vi "Handle timeline menu options.vi"(6 "Xinformation In":T2, 7 "Waveform Ref in":T1, 9 "ItemTag":string, 11 "Timeline Ref in":T4) -> (0 "error out":errorcluster, 3 "Timeline Ref out":T4, 4 "Xinformation Out":T2)   [LabVIEW 2020, in "XGrapher.xctl"]
uses:
  XGrapher.xctl
  Typedefs/Xctrl-Timeline graph ref.ctl
  Typedefs/Xinformation.ctl
  Typedefs/Xcrtl-Click Operation.ctl
  Typedefs/Xctrl-Waveform graph ref.ctl
  Typedefs/Registered event names enum.ctl
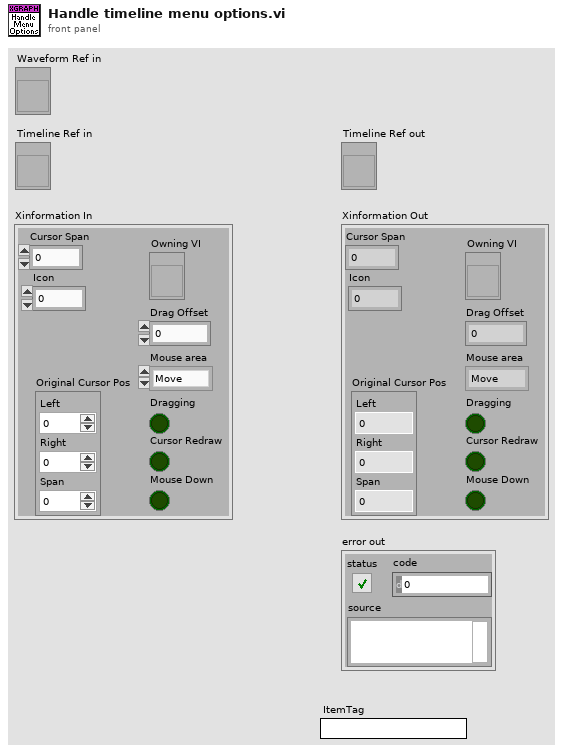
[diagram p1: front panel]
types:
  T1 = typedef "XGrapher.xctl/Xctrl-Waveform graph ref.ctl" = refnum<vi>
  T2 = typedef "XGrapher.xctl/Xinformation.ctl" = cluster{"Cursor Span":dbl, "Icon":u16, "Mouse Down":bool, "Owning VI":refnum<vi>, "Mouse area":T3, "Dragging":bool, "Drag Offset":dbl, "Original Cursor Pos":cluster{"Left":dbl, "Right":dbl, "Span":dbl}, "Cursor Redraw":bool}
  T3 = typedef "XGrapher.xctl/Xcrtl-Click Operation.ctl" = enum16{"Move", "left cursor", "right cursor", "none"}
  T4 = typedef "XGrapher.xctl/Xctrl-Timeline graph ref.ctl" = refnum<vi>
  T5 = typedef "Registered event names enum.ctl" = enum16{"Register", "Load dataset in funct viewer", "Re-process data", "Export selected ROI data-full"}
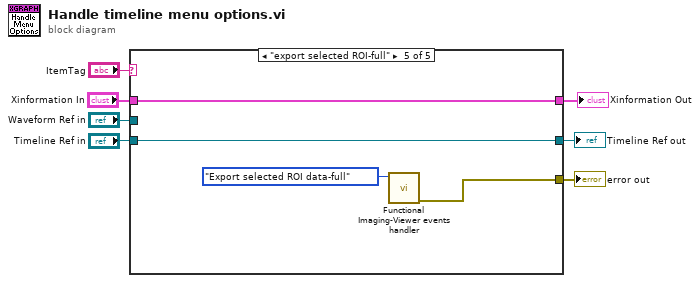
[diagram p0: block diagram]
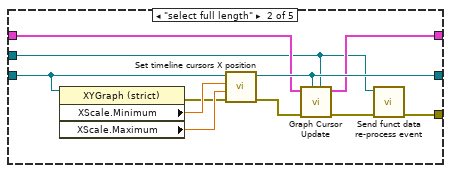
[diagram p3: hidden frame]
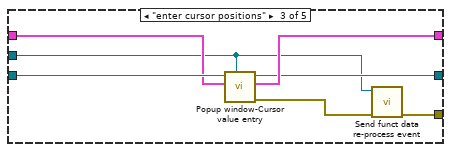
[diagram p4: hidden frame]
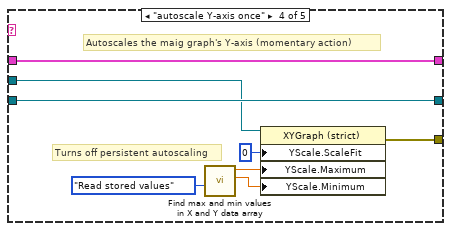
[diagram p5: hidden frame]
diagram:
  n1 = case shown="\"export selected ROI-full\"" "ItemTag" {
    tunnel: [_ w14 w21 w30 w36] -> w5
    tunnel: "Timeline Ref in" -> [w9 w13 w27 w34 w38]
    tunnel: [w9 w19 w24 w34 w38] -> w7
    tunnel: "Waveform Ref in" -> [_ w16 w23 w32 _]
    tunnel: "Xinformation In" -> [w8 w18 w26 w35 w39]
    tunnel: [w8 w17 w25 w35 w39] -> w1
    frame Default {
    }
    frame "select full length" {
      n2 = property on="Property Node" class="XYGraph (strict)"(reference=w13) -> (error out=w10:errorcluster, "XScale.Minimum"=w12:dbl, "XScale.Maximum"=w11:dbl)  [unwired: 1 in, 1 out]
      n3 = call "Set timeline cursors X position.vi"("error in (no error)"=w10, "Right"=w11, "Left"=w12, "Timeline Graph in"=w13) -> ("error out"=w20:errorcluster, "Timeline Graph out"=w19:T4)  [unwired: 6 in]
      n4 = call "Graph Cursor Update.vi"("Waveform Ref in"=w16, "Timeline Ref in"=w19, "error in (no error)"=w20, "Xinformation In"=w18) -> ("error out"=w15:errorcluster, "Xinformation Out"=w17:T2)  [unwired: 5 in, 1 out]
      n5 = call "Send funct data re-process event.vi"("error in (no error)"=w15, "Waveform Graph in"=w16) -> ("error out"=w14:errorcluster)  [unwired: 9 in]
    }
    frame "enter cursor positions" {
      n6 = call "Popup window-Cursor value entry.vi"("Waveform Ref in"=w23, "Xinformation In"=w26, "Timeline Ref in"=w27) -> ("error out"=w22:errorcluster, "Xinformation Out"=w25:T2, "Timeline Ref out"=w24:T4)  [unwired: 5 in, 1 out]
      n7 = call "Send funct data re-process event.vi"("error in (no error)"=w22, "Waveform Graph in"=w23) -> ("error out"=w21:errorcluster)  [unwired: 9 in]
    }
    frame "autoscale Y-axis once" {
      # "Turns off persistent autoscaling"
      # "Autoscales the maig graph's Y-axis (momentary action)"
      n8 = call "Find max and min values in X and Y data array.vi"("Function"=enum16{"Analyse & store", "Read stored values"}."Read stored values") -> ("Min intensity among all datasets"=w31:dbl, "Max intensity among all datasets"=w29:dbl)  [unwired: 6 in, 3 out]
      n9 = property on="Property Node" class="XYGraph (strict)"(reference=w32, "YScale.ScaleFit"=u8 0 ("Y Scale.Scale Fit"), "YScale.Maximum"=w29, "YScale.Minimum"=w31) -> (error out=w30:errorcluster)  [unwired: 1 in, 1 out]
    }
    frame "export selected ROI-full" {
      n10 = call "Functional Imaging-Viewer events handler.vi"("Event Function"=Registered_event_names_enum."Export selected ROI data-full") -> ("error out"=w36:errorcluster)  [unwired: 9 in, 1 out]
    }
  }
  "Timeline Ref out" <- w7
  "error out" <- w5
  "Xinformation Out" <- w1
